vi "getRfChannelSafeStates.vi"(8 "error in (no error)":errorcluster, 10 "deviceName":string, 11 "deviceDataBase in":refnum<class "deviceDataBase.lvclass">) -> (0 "error out":errorcluster, 1 "safestates":T1(array[cluster])=[{"Frequency(MHz)"=100.0, "Amplitude"=1.0, "Phase"=0.0, "OutputForm"=enum."Sine"}, {"Frequency(MHz)"=100.0, "Amplitude"=1.0, "Phase"=0.0, "OutputForm"=enum."Sine"}], 2 "ChannelAddresses":string[](array[string]), 3 "deviceDataBase out":refnum<class "deviceDataBase.lvclass">)   [LabVIEW 2009, in "Tools.lvlib" / "DatabaseHelpers.lvlib" / "deviceDataBase.lvclass"]
uses:
  deviceDataBase.lvclass
  deviceDataBase.lvclass/deviceDataBase.ctl
  Database Objects/Channel/Channel.lvclass
  Database Objects/DeviceArray/DeviceArray.lvclass
  Database Objects/device/device.lvclass
  Database Objects/ChannelArray/ChannelArray.lvclass
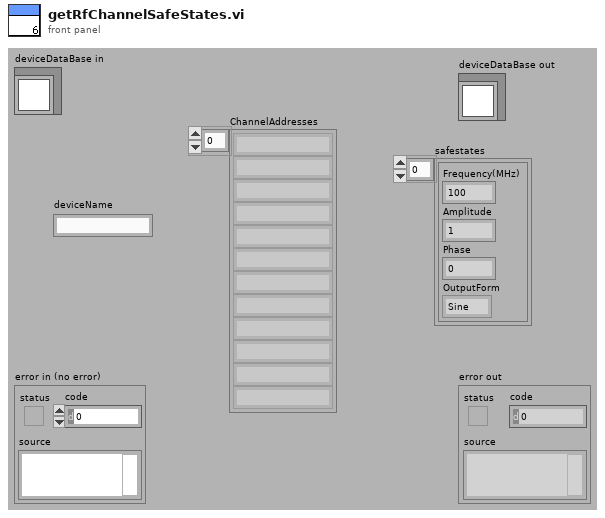
[diagram p1: front panel]
types:
  T1 = cluster{"Frequency(MHz)":dbl, "Amplitude":dbl, "Phase":dbl, "OutputForm":enum16{"Sine", "Square", "Triangle", "Arbitrary"}}[]
  T2 = cluster{"Frequency(MHz)":dbl, "Amplitude":dbl, "Phase":dbl, "OutputForm":enum16{"Sine", "Square", "Triangle", "Arbitrary"}}
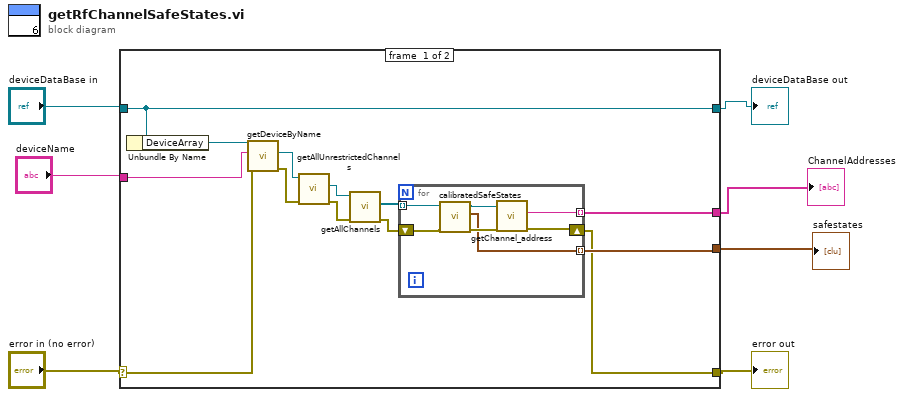
[diagram p0: block diagram]
diagram:
  n1 = case shown="No Error" "error in (no error)" {
    selector: "error in (no error)" -> [w17 w29]
    tunnel: [w8 w29] -> w5
    tunnel: [w20 w28] -> w6
    tunnel: "deviceDataBase in" -> [w20 w28]
    tunnel: "deviceName" -> [w18 _]
    tunnel: [w10 _] -> w1
    tunnel: [w9 _] -> w2
    frame #0 {
      n2 = Unbundle By Name(w20) -> ("DeviceArray"=w19:refnum<class "DeviceArray.lvclass">)
      n3 = call "getDeviceByName.vi"("error in (no error)"=w17, "deviceName"=w18, "DeviceArray in"=w19) -> ("error out"=w15:errorcluster, "device.lvclass"=w16:refnum<class "device.lvclass">)  [unwired: 5 in, 2 out]
      n4 = call "getAllUnrestrictedChannels.vi"("error in (no error)"=w15, "device in"=w16) -> ("error out"=w13:errorcluster, "ChannelArray.lvclass"=w14:refnum<class "ChannelArray.lvclass">)  [unwired: 7 in, 1 out]
      n5 = call "getAllChannels.vi"("error in (no error)"=w13, "ChannelArray.lvclass in"=w14) -> ("error out"=w12:errorcluster, "channels"=w11:refnum<class "Channel.lvclass">[])  [unwired: 7 in, 1 out]
      n6 = for {
        shift-right: [w26] -> w8
        shift-left: w12 -> [w24]
        tunnel: w11 -> [w25] mode=indexing
        tunnel: [w21] -> w9 mode=indexing
        tunnel: [w27] -> w10 mode=indexing
        n7 = call-dynamic "calibratedSafeStates.vi"("error in (no error)"=w24, "Channel in"=w25) -> ("error out"=w22:errorcluster, "OutputDefaults"=w21:T2, "Channel out"=w23:refnum<class "Channel.lvclass">)  [unwired: 7 in]
        n8 = call "getChannel_address.vi"("error in (no error)"=w22, "Channel.lvclass in"=w23) -> ("error out"=w26:errorcluster, "channel_address"=w27:string)  [unwired: 7 in, 1 out]
      }
    }
    frame #1 {
    }
  }
  "error out" <- w5
  "deviceDataBase out" <- w6
  "safestates" <- w2
  "ChannelAddresses" <- w1
